vi "Stage tester - live move.vi"() -> ()   [LabVIEW 2017]
panel:
  out "Loop":i32
  in  "stop":bool
  in  "Z":dbl
  in  "Y":dbl
  in  "X":dbl
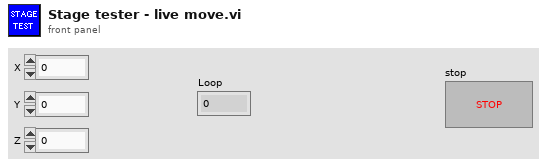
[diagram p1: front panel]
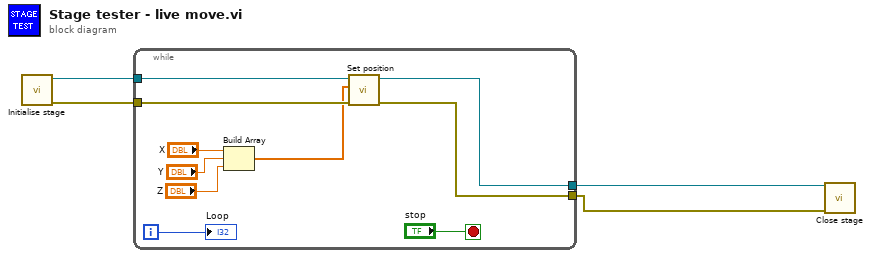
[diagram p0: block diagram]
diagram:
  n1 = call "Initialise stage.vi"() -> ("error out"=w3:errorcluster, "Stage VISA reference"=w2:refnum<visa-resource-name>)  [unwired: 10 in]
  n2 = while {
    tunnel: w3 -> [w13]
    tunnel: [w12] -> w4
    tunnel: w2 -> [w10]
    tunnel: [w11] -> w1
    i -> [w5]
    stop <- "stop" stop-if-true
    n3 = Build Array("X", "Y", "Z") -> (w6:dbl[])
    n4 = call "Set position.vi"("error in"=w13, "Set stage position"=w6, "Stage VISA in"=w10) -> ("error out"=w12:errorcluster, "Stage VISA out"=w11:refnum<visa-resource-name>)  [unwired: 7 in]
    "Loop" <- w5
  }
  n5 = call "Close stage.vi"("error in"=w4, "VISA resource name"=w1) -> ()  [unwired: 9 in, 1 out]
